vi "SetState.vi"(8 "error in (no error)":errorcluster, 10 "State":T1) -> (0 "error out":errorcluster)   [LabVIEW 2019, in "MainStates.lvclass"]
uses:
  MainStates.lvclass
  TypeDef/MainState.ctl
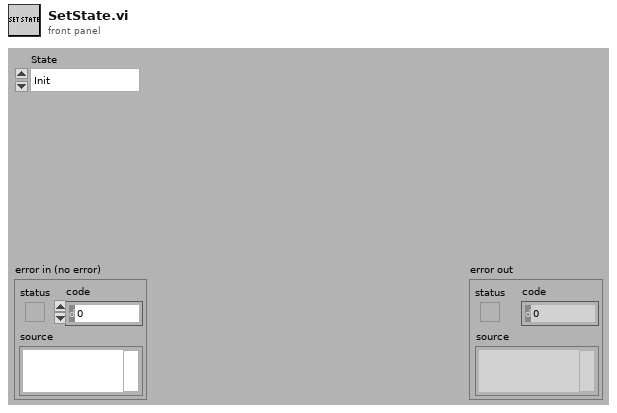
[diagram p1: front panel]
types:
  T1 = typedef "MainState.ctl" = enum16{"Init", "Idle", "Safe Stop", "Normal Working", "Critical Error", "Closing"}
  T2 = typedef "MainStates.lvclass/ObjectAttributes.ctl" = cluster{"State":T3}
  T3 = typedef "MainStates.lvclass/MainState.ctl" = enum16{"Init", "Idle", "Safe Stop", "Normal Working", "Critical Error", "Closing"}
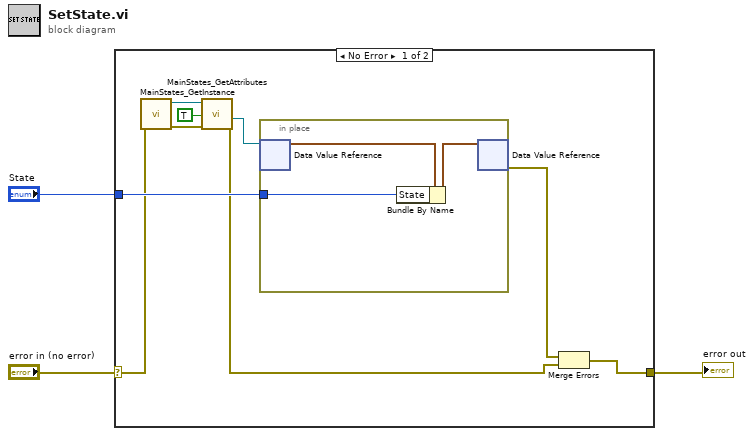
[diagram p0: block diagram]
diagram:
  n1 = case shown="No Error" "error in (no error)" {
    selector: "error in (no error)" -> [w6 w16]
    tunnel: [w10 w16] -> w2
    tunnel: "State" -> [w12 _]
    frame No Error {
      n2 = call "MainStates_GetInstance.vi"("error in (no error)"=w6) -> ("error out"=w8:errorcluster, "reference out"=w7:refnum<class "MainStates.lvclass">)  [unwired: 6 in, 3 out]
      n3 = call "MainStates_GetAttributes.vi"("error in (no error)"=w8, "OnlyGetDvrReference(False)"=TRUE, "reference in"=w7) -> ("error out"=w9:errorcluster, "DataRef"=w5:refnum<data-value>)  [unwired: 5 in, 2 out]
      n4 = in-place {
        in-place-border: w12 -> [w15]
        n5 = in-place-dvr #1(w5) -> (w14:T2)  [unwired: 1 out]
        n6 = Bundle By Name(cluster=w14, "State"=w15) -> (w13:T2)
        n7 = in-place-dvr #1(w13) -> (w11:errorcluster)  [unwired: 1 out]
      }
      n8 = Merge Errors(w11, w9) -> (w10:errorcluster)
    }
    frame Error {
    }
  }
  "error out" <- w2
